vi "Real_time_success.vi"() -> ()   [LabVIEW 2018]
uses:
  <vilib>/Analysis/_algsub.llb/Vector Norm.vi
  <vilib>/Analysis/_algsub.llb/Real Vector Norm.vi
  <vilib>/Analysis/baseanly.llb/Outer Product.vi
  <vilib>/Analysis/baseanly.llb/Real Outer Product.vi
  <vilib>/robotics/Kinematics/Create Lie Group Matrix.vi
  <vilib>/Analysis/baseanly.llb/Real Inverse Matrix.vi
  <vilib>/imath/engines/lvmath2/RunTimeEngine/NodeEndStatement/NIMS_NodeEndStatement_Output.vi
  <instcachedir>/0/NIMS_NodeEndStatement_Output_53EC0D466D134D7ABD903AC30B43404B.lvgen/NIMS_NodeEndStatement_Output_53EC0D466D134D7ABD903AC30B43404B_005.vi
  <instcachedir>/0/NIMS_NodeEndStatement_Output_53EC0D466D134D7ABD903AC30B43404B.lvgen/NIMS_NodeEndStatement_Output_53EC0D466D134D7ABD903AC30B43404B_000.vi
  <instcachedir>/0/NIMS_NodeEndStatement_Output_53EC0D466D134D7ABD903AC30B43404B.lvgen/NIMS_NodeEndStatement_Output_53EC0D466D134D7ABD903AC30B43404B_002.vi
  <vilib>/imath/engines/lvmath2/RunTimeEngine/ErrorHandling/NIMS_Finalize Error.vi
  <vilib>/Analysis/Matrix/Numeric/Conversions/Matrix To Array - RM.vi
  <vilib>/imath/engines/lvmath2/RunTimeEngine/IndexRead/NIMS M(S,S).vi
  <instcachedir>/0/NIMS M(S,S)_AC51E74150A542F7991B9634C66F3096.lvgen/NIMS M(S,S)_AC51E74150A542F7991B9634C66F3096_000.vi
  <vilib>/imath/engines/lvmath2/RunTimeEngine/BuiltInFunctions/abs/NIMS_abs(signed).vi
  <instcachedir>/0/NIMS_abs(signed)_C4FCB8E6058B49B797C7C8D53CA5F6EC.lvgen/NIMS_abs(signed)_C4FCB8E6058B49B797C7C8D53CA5F6EC_000.vi
  <vilib>/imathl/engines/lvmath/Functions/Error Handling/Create Error.vi
  <vilib>/imath/engines/lvmath2/RunTimeEngine/BuiltInFunctions/atan2/NIMS_atan2.vi
  <instcachedir>/0/NIMS_atan2_A91AA4A7D42247EDBE8F76DB99AF04A4.lvgen/NIMS_atan2_A91AA4A7D42247EDBE8F76DB99AF04A4_002.vi
  <vilib>/imath/engines/lvmath2/RunTimeEngine/ErrorHandling/NIMS_Create Error From Enums.vi
  <vilib>/imath/engines/lvmath2/RunTimeEngine/BuiltInFunctions/cos/NIMS_cos(C).vi
  <instcachedir>/0/NIMS_cos(C)_96B8A70E6B8E4D29AD8526A89C8CF3DF.lvgen/NIMS_cos(C)_96B8A70E6B8E4D29AD8526A89C8CF3DF_001.vi
  <instcachedir>/0/NIMS_atan2_A91AA4A7D42247EDBE8F76DB99AF04A4.lvgen/NIMS_atan2_A91AA4A7D42247EDBE8F76DB99AF04A4_001.vi
  <vilib>/imath/engines/lvmath2/RunTimeEngine/IndexRead/NIMS V(S).vi
  <instcachedir>/0/NIMS V(S)_0488751826AF41519A22953C041130DC.lvgen/NIMS V(S)_0488751826AF41519A22953C041130DC_003.vi
  <vilib>/imath/engines/lvmath2/RunTimeEngine/BuiltInFunctions/sin/NIMS_sin(C).vi
  <instcachedir>/0/NIMS_sin(C)_7FE83C8DCD97403BBE687635FA1F837E.lvgen/NIMS_sin(C)_7FE83C8DCD97403BBE687635FA1F837E_001.vi
  <instcachedir>/0/NIMS V(S)_0488751826AF41519A22953C041130DC.lvgen/NIMS V(S)_0488751826AF41519A22953C041130DC_000.vi
  <vilib>/imath/engines/lvmath2/RunTimeEngine/ArithmeticOperatorToken/NIMS_ArithmeticOperator_multmx.vi
  <instcachedir>/0/NIMS_ArithmeticOperator_multmx_622CA76F9646436AB036D42A9A1CE0E6.lvgen/NIMS_ArithmeticOperator_multmx_622CA76F9646436AB036D42A9A1CE0E6_004.vi
  <vilib>/imath/engines/lvmath2/RunTimeEngine/ArithmeticOperatorToken/NIMS_ArithmeticOperator_multmx(M,CV).vi
  <instcachedir>/0/NIMS_ArithmeticOperator_multmx(M,CV)_2F1CD6A2FE4F4213A4AD1C901C2750F5.lvgen/NIMS_ArithmeticOperator_multmx(M,CV)_2F1CD6A2FE4F4213A4AD1C901C2750F5_000.vi
  <vilib>/imath/engines/lvmath2/RunTimeEngine/ArithmeticOperatorToken/NIMS_ArithmeticOperator_multmx(M,CV)-internal.vi
  <instcachedir>/0/NIMS_ArithmeticOperator_multmx(M,CV)-internal_5287250D8D1D4A3E9F77F5DF08D432E0.lvgen/NIMS_ArithmeticOperator_multmx(M,CV)-internal_5287250D8D1D4A3E9F77F5DF08D432E0_004.vi
  <vilib>/imath/engines/lvmath2/RunTimeEngine/ArithmeticOperatorToken/NIMS_ArithmeticOperator_minus.vi
  <instcachedir>/0/NIMS_ArithmeticOperator_minus_C4D0373119CC411691B2E50DF2E09F22.lvgen/NIMS_ArithmeticOperator_minus_C4D0373119CC411691B2E50DF2E09F22_009.vi
  <instcachedir>/0/NIMS_ArithmeticOperator_multmx_622CA76F9646436AB036D42A9A1CE0E6.lvgen/NIMS_ArithmeticOperator_multmx_622CA76F9646436AB036D42A9A1CE0E6_008.vi
  <vilib>/imath/engines/lvmath2/RunTimeEngine/IndexRead/NIMS M(S).vi
  <instcachedir>/0/NIMS M(S)_B826C018497E4940AE96BD27B540B6FB.lvgen/NIMS M(S)_B826C018497E4940AE96BD27B540B6FB_004.vi
  <vilib>/imath/engines/lvmath2/RunTimeEngine/Managers/WorkSpace/UID Generator.vi
  <vilib>/imath/engines/lvmath2/RunTimeEngine/RunTimeType/NIMS_RunTimeType_From StrictType (excl LVString).vi
  <instcachedir>/0/NIMS_RunTimeType_From StrictType (excl LVString)_E7E34A65C99947108168652BAD14964D.lvgen/NIMS_RunTimeType_From StrictType (excl LVString)_E7E34A65C99947108168652BAD14964D_000.vi
  <vilib>/imath/engines/lvmath2/RunTimeEngine/LocalVariableDefStatement/MC_LocalVariableDefStatement_Display.vi
  <instcachedir>/0/NIMS M(S)_B826C018497E4940AE96BD27B540B6FB.lvgen/NIMS M(S)_B826C018497E4940AE96BD27B540B6FB_000.vi
  <vilib>/imath/engines/lvmath2/RunTimeEngine/Managers/SymbolTable/Clear UID.vi
  <vilib>/Analysis/Matrix/Numeric/Multiply/Multiply.vi
  <vilib>/Analysis/Matrix/Numeric/Multiply/Multiply - RM,R.vi
  <vilib>/Analysis/Matrix/Numeric/Multiply/Multiply - R,RM.vi
  <vilib>/Analysis/Matrix/Numeric/Add/Add.vi
  <vilib>/Analysis/Matrix/Numeric/Add/Add - RM,RM.vi
  <instcachedir>/0/NIMS_NodeEndStatement_Output_53EC0D466D134D7ABD903AC30B43404B.lvgen/NIMS_NodeEndStatement_Output_53EC0D466D134D7ABD903AC30B43404B_001.vi
  <instcachedir>/0/NIMS_NodeEndStatement_Output_53EC0D466D134D7ABD903AC30B43404B.lvgen/NIMS_NodeEndStatement_Output_53EC0D466D134D7ABD903AC30B43404B_008.vi
  <vilib>/imath/engines/lvmath2/RunTimeEngine/IndexRead/NIMS M($,S).vi
  <instcachedir>/0/NIMS M($,S)_3E5749BBB62E49528D4765A77F1F6D98.lvgen/NIMS M($,S)_3E5749BBB62E49528D4765A77F1F6D98_000.vi
  <vilib>/imath/engines/lvmath2/RunTimeEngine/RowToken/NIMS_RowToken_SorRV_CV.vi
  <instcachedir>/0/NIMS_RowToken_SorRV_CV_E9A223509C5746E8B9F22970C86A52C1.lvgen/NIMS_RowToken_SorRV_CV_E9A223509C5746E8B9F22970C86A52C1_000.vi
  <vilib>/Analysis/NI_AALBase.lvlib
  <vilib>/gmath/NI_Gmath.lvlib
  <vilib>/Analysis/Matrix/NI_Matrix.lvlib
  <vilib>/robotics/Kinematics/NI_Kinematics.lvlib
  <vilib>/imath/engines/lvmath2/RunTimeEngine/Managers/SymbolTable/NIMS_WorkSpace.lvlib
panel:
  out "Yaw":cluster{"E1_now":dbl[], "t_now":dbl[]}(graph)
  out "Pitch":cluster{"E1_now":dbl[], "t_now":dbl[]}(graph)
  out "Roll":cluster{"E1_now":dbl[], "t_now":dbl[]}(graph)
  in  "MOI(kg*m^2)":dbl[][](array[numeric])
  in  "COG(m)":dbl[](array[numeric])
  in  "Mass (kg)":dbl
  in  "Simulation Time(sec)":dbl
  # "Physical Parameters"
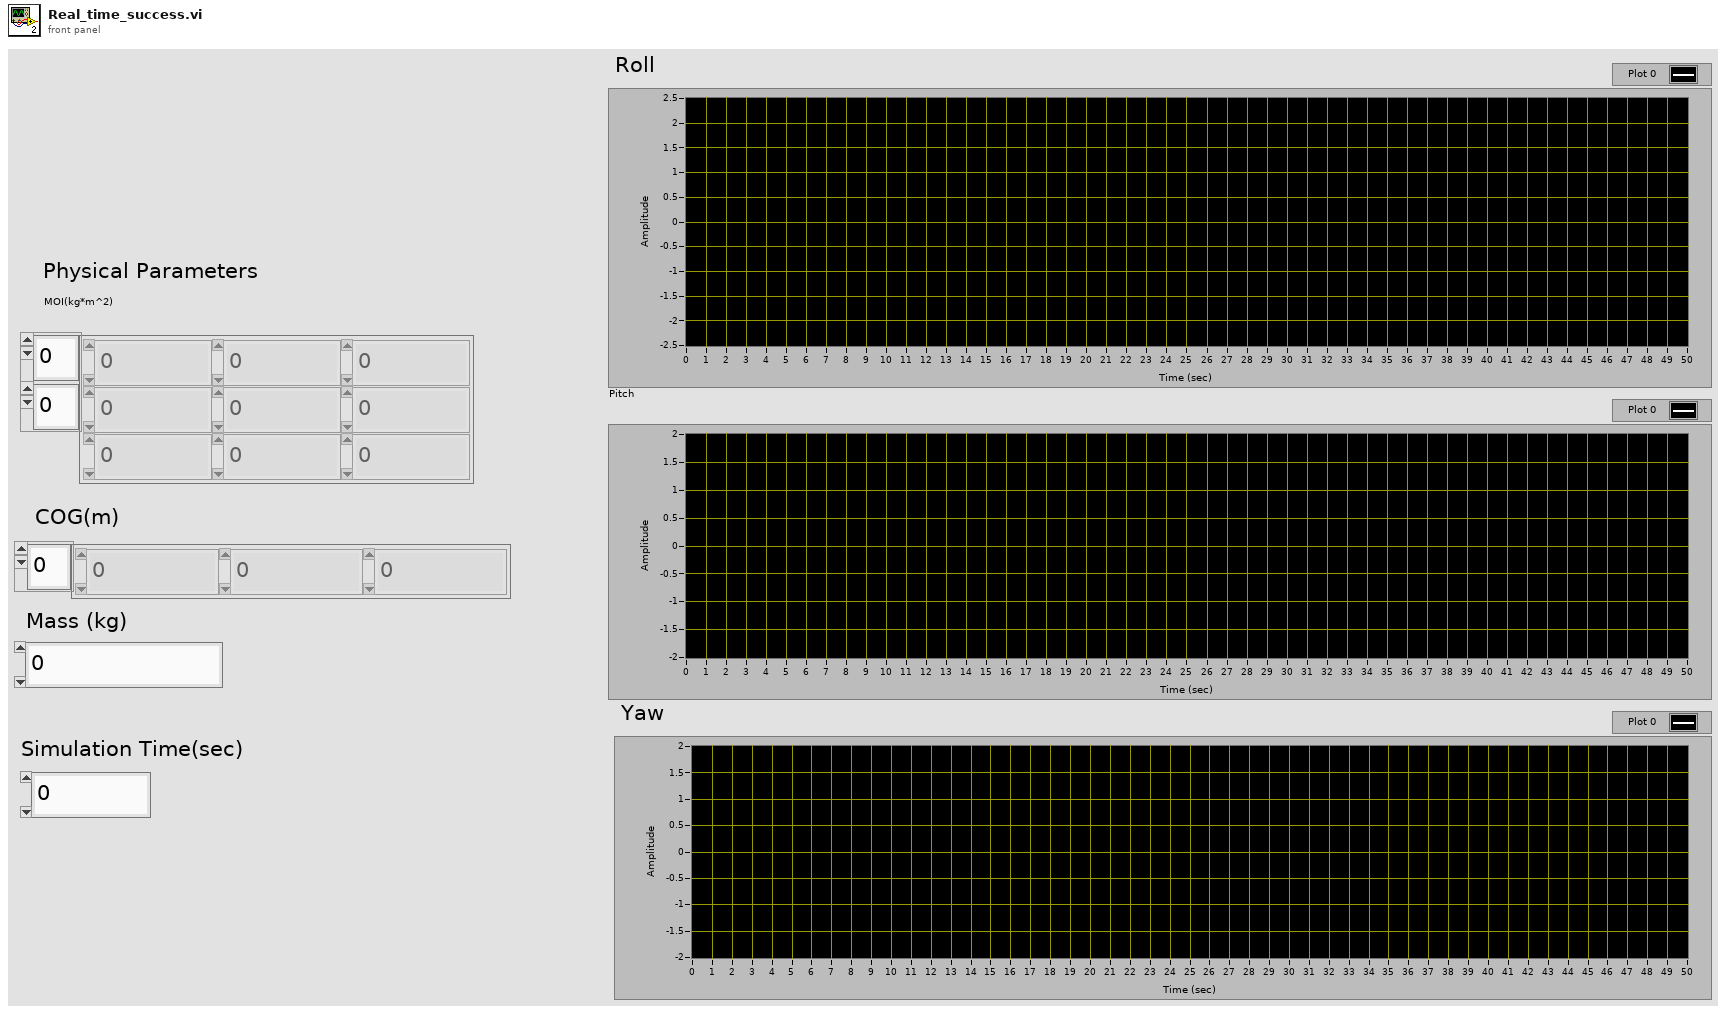
[diagram p1: front panel]
types:
  T1 = cluster{"E1":cdb[], "E2":dbl[], "E3":dbl[], "t":dbl[]}
  T2 = typedef "NI_Matrix.lvlib/RealMatrix.ctl" = dbl[][]
  T3 = typedef "NI_Kinematics.lvlib/Quaternion.ctl" = dbl[]
  T4 = cluster{"E1_now":cdb[], "E2_now":cdb[], "E3_now":dbl[], "t_now":dbl[]}
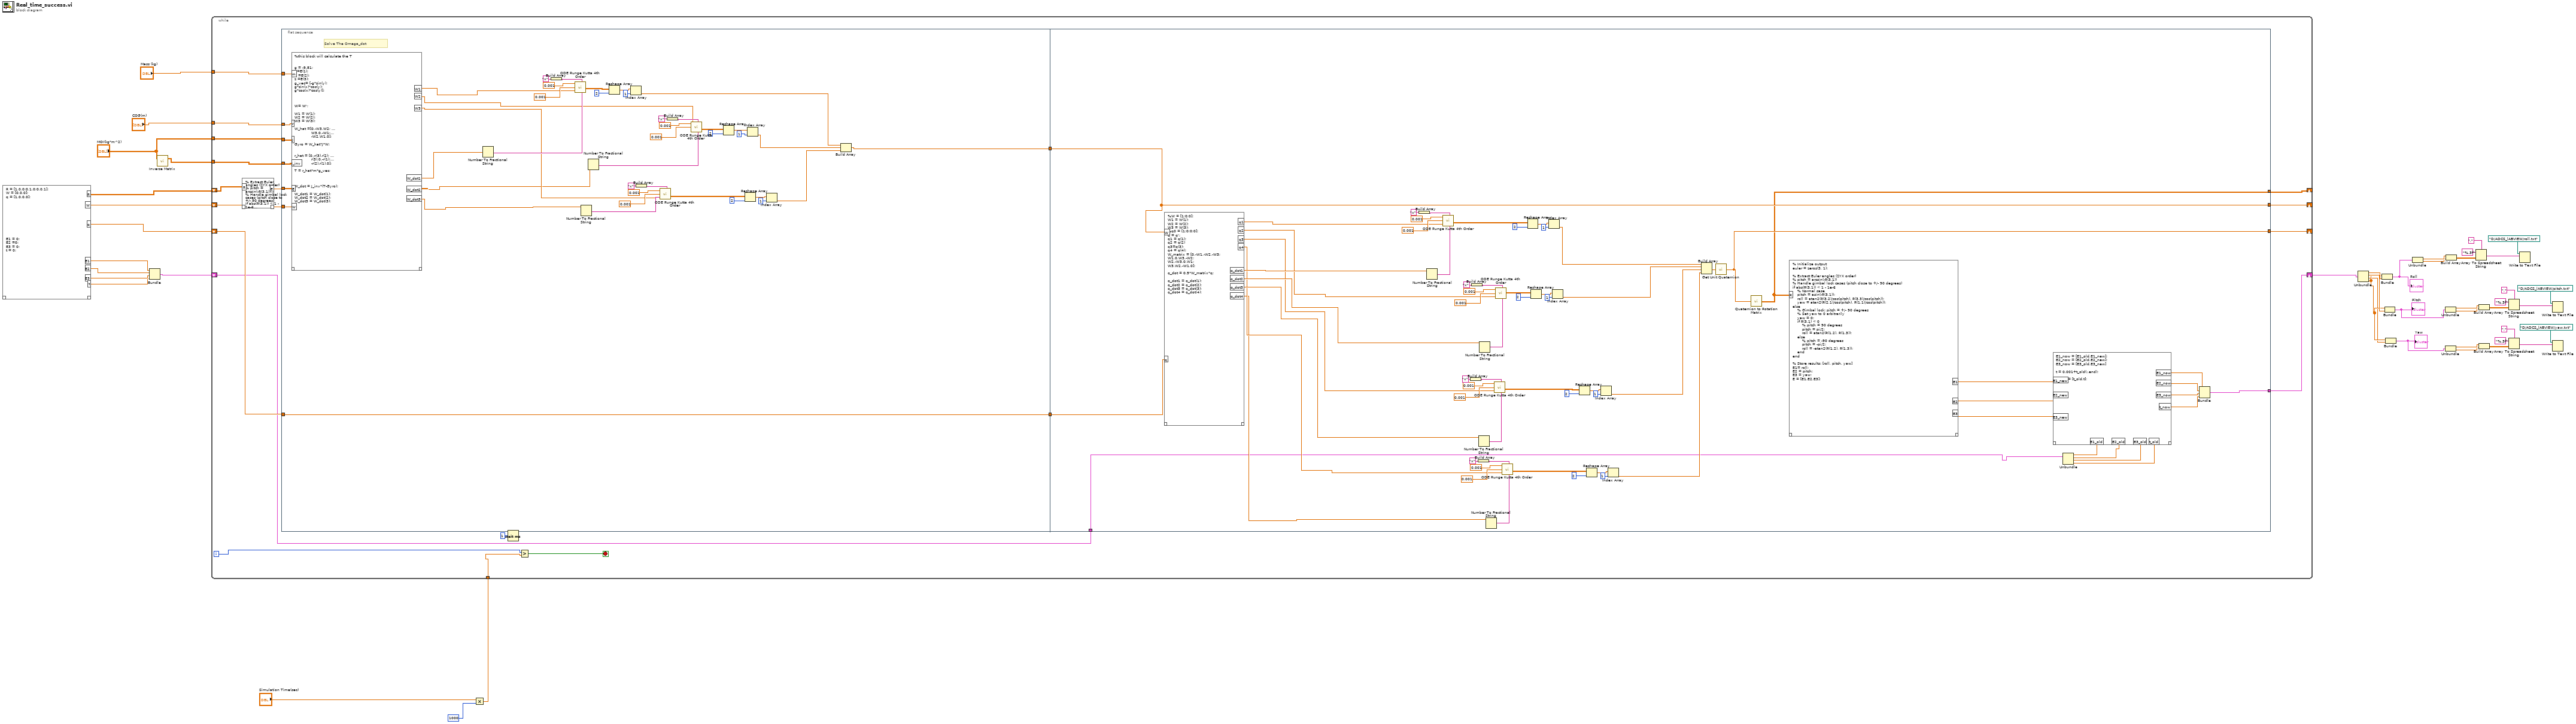
[diagram p0: block diagram]
diagram:
  n1 = mathscript code="R = [1,0,0;0,1,0;0,0,1];\nW = [0,0,0];\nq = [1,0,0,0];\n\n\n\n\n\n\n\n\n\n\nE1 = 0;\nE2 =0;\nE3 = 0;\nt = 0;"() -> ("R"=w37:dbl[][], "W"=w36:dbl[], "q"=w35:dbl[], "E1"=w34:cdb[], "E2"=w33:dbl[], "E3"=w32:dbl[], "t"=w30:dbl[])  [unwired: 1 in, 1 out]
  n2 = Bundle("E1"=w34, "E2"=w33, "E3"=w32, "t"=w30) -> (w31:T1)  [unwired: 1 in]
  n3 = call-poly <vilib>:"Inverse Matrix.vi"("Input Matrix"="MOI(kg*m^2)") -> ("Inverse Matrix"=w39:T2)  [unwired: 1 in, 1 out]
  n4 = Multiply(x="Simulation Time(sec)", y=1000) -> (x*y=w42:dbl)
  n5 = while {
    tunnel: w42 -> [w49]
    tunnel: "Mass (kg)" -> [w59]
    tunnel: "COG(m)" -> [w60]
    tunnel: w39 -> [w62]
    tunnel: "MOI(kg*m^2)" -> [w61]
    shift-right: [w52] -> _
    shift-left: w37 -> [w57]
    shift-right: [w51] -> _
    shift-left: w36 -> [w58]
    shift-right: [w53] -> _
    shift-left: w35 -> [w54]
    shift-right: [w46] -> w29
    shift-left: w31 -> [w47]
    i -> [w48]
    stop <- w50 stop-if-true
    n6 = mathscript code="% Extract Euler angles (ZYX order)\n% pitch = arcsin(-R(3,1))\n% Handle gimbal lock cases (pitch close to +/- 90 degrees)\nif abs(R(3,1)) < 1 - 1e-6\n    % Normal case\n    pitch = asin(-R(3,1));\n    roll = atan2(R(3,2)/cos(pitch), R(3,3)/cos(pitch));\n    yaw = atan2(R(2,1)/cos(pitch), R(1,1)/cos(pitch));\nelse\n    % Gimbal lock: pitch = +/- 90 degrees\n    % Set yaw to 0 arbitrarily\n    yaw = 0;\n    if R(3,1) < 0\n        % pitch = 90 degrees\n        pitch = pi/2;\n        roll = atan2(R(1,2), R(1,3));\n    else\n        % pitch = -90 degrees\n        pitch = -pi/2;\n        roll = -atan2(R(1,2), R(1,3));\n    end\nend\n\n% Store results: [roll, pitch, yaw]\nE1= roll;\nE2 = pitch;\nE3 = yaw;\nE = [E1,E2,E3];"("R"=w57) -> ("E"=w56:cdb[])  [unwired: 1 in, 1 out]
    n7 = flat-sequence {
      tunnel: w56 -> [w383]
      tunnel: w62 -> [w382]
      tunnel: w61 -> [w381]
      tunnel: w60 -> [w380]
      tunnel: w59 -> [w379]
      tunnel: w58 -> [w378]
      tunnel: [w341] -> w55
      tunnel: w54 -> [w341]
      tunnel: [w340] -> w45
      tunnel: w55 -> [w803]
      tunnel: [w802] -> w53
      tunnel: [w800] -> w52
      tunnel: [w801] -> w51
      tunnel: w47 -> [w793]
      tunnel: [w789] -> w46
      tunnel: w45 -> [w801]
      frame #0 {
        # "Solve The Omega_dot"
        n8 = mathscript code="%this block will calculate the T\n\n\ng = -9.81;\nx=E(1);\ny =E(2);\nz =E(3);\ng_vec= [-g*sin(y);\ng*sin(x)*cos(y);\ng*cos(x)*cos(y)];\n\n\n\nW= W';\n\nW1 = W(1);\nW2 = W(2);\nW3 = W(3);\n\nW_hat =[0,-W3,W2; ...\n              W3,0,-W1;...\n              -W2,W1,0];\n\nGyro = W_hat*J*W;\n\n\nr_hat = [0,-r(3),r(2); ...\n              r(3),0,-r(1);...\n              -r(2),r(1),0];\n\nT = r_hat*m*g_vec;\n\n\n\nW_dot = J_inv*(T-Gyro);\n\nW_dot1 = W_dot(1);\nW_dot2 = W_dot(2);\nW_dot3 = W_dot(3);"("E"=w383, "J"=w381, "J_inv"=w382, "r"=w380, "m"=w379, "W"=w378) -> ("W_dot1"=w342:dbl[], "W_dot2"=w343:dbl[], "W_dot3"=w344:dbl[], "W1"=w347:dbl[], "W2"=w346:dbl[], "W3"=w345:dbl[])  [unwired: 1 in, 1 out]
        n9 = Number To Fractional String(number=w342) -> (F-format string=w373:string[])  [unwired: 3 in]
        n10 = Build Array("x") -> (w376:string[])
        n11 = call <vilib>:"ODE Runge Kutta 4th Order.vi"("time end"=0.001, "h (step rate)"=0.001, "X0"=w347, "X (name of variables)"=w376, "F(X,t) (right sides of the ODE\nas functions of X and t)"=w373) -> ("X Values (solution)"=w369:dbl[][])  [unwired: 2 in, 3 out]
        n12 = Number To Fractional String(number=w344) -> (F-format string=w355:string[])  [unwired: 3 in]
        n13 = Number To Fractional String(number=w343) -> (F-format string=w364:string[])  [unwired: 3 in]
        n14 = Reshape Array(w369, 2 ("dimension size")) -> (w371:dbl[])
        n15 = Index Array(array=w371, index=1) -> (element=w350:dbl)
        n16 = Build Array("x") -> (w358:string[])
        n17 = call <vilib>:"ODE Runge Kutta 4th Order.vi"("time end"=0.001, "h (step rate)"=0.001, "X0"=w345, "X (name of variables)"=w358, "F(X,t) (right sides of the ODE\nas functions of X and t)"=w355) -> ("X Values (solution)"=w351:dbl[][])  [unwired: 2 in, 3 out]
        n18 = Build Array("x") -> (w367:string[])
        n19 = call <vilib>:"ODE Runge Kutta 4th Order.vi"("time end"=0.001, "h (step rate)"=0.001, "X0"=w346, "X (name of variables)"=w367, "F(X,t) (right sides of the ODE\nas functions of X and t)"=w364) -> ("X Values (solution)"=w360:dbl[][])  [unwired: 2 in, 3 out]
        n20 = Reshape Array(w360, 2 ("dimension size")) -> (w362:dbl[])
        n21 = Reshape Array(w351, 2 ("dimension size")) -> (w353:dbl[])
        n22 = Index Array(array=w362, index=1) -> (element=w349:dbl)
        n23 = Index Array(array=w353, index=1) -> (element=w348:dbl)
        n24 = Build Array(w350, w349, w348) -> (w340:dbl[])
      }
      frame #1 {
        n25 = mathscript code="%W = [1;0;0];\nW1 = W(1);\nW2 = W(2);\nW3 = W(3);\n%q0 = [1;0;0;0];\nq = q';\nq1 = q(1);\nq2 = q(2)\nq3=q(3);\nq4 = q(4);\nW_matrix = [0,-W1,-W2,-W3;\nW1,0,W3,-W2;\nW2,-W3,0,W1;\nW3,W2,-W1,0];\n\nq_dot = 0.5*W_matrix*q;\n\nq_dot1 = q_dot(1);\nq_dot2 = q_dot(2);\nq_dot3 = q_dot(3);\nq_dot4 = q_dot(4);"("q"=w803, "W"=w801) -> ("q_dot1"=w842:dbl[], "q_dot2"=w831:dbl[], "q_dot3"=w820:dbl[], "q_dot4"=w809:dbl[], "q1"=w843:dbl[], "q2"=w832:dbl[], "q3"=w821:dbl[], "q4"=w810:dbl[])  [unwired: 1 in, 1 out]
        n26 = Build Array("x") -> (w851:string[])
        n27 = Number To Fractional String(number=w842) -> (F-format string=w848:string[])  [unwired: 3 in]
        n28 = call <vilib>:"ODE Runge Kutta 4th Order.vi"("time end"=0.001, "h (step rate)"=0.001, "X0"=w843, "X (name of variables)"=w851, "F(X,t) (right sides of the ODE\nas functions of X and t)"=w848) -> ("X Values (solution)"=w844:dbl[][])  [unwired: 2 in, 3 out]
        n29 = Build Array("x") -> (w829:string[])
        n30 = Build Array("x") -> (w840:string[])
        n31 = Build Array("x") -> (w818:string[])
        n32 = Number To Fractional String(number=w820) -> (F-format string=w826:string[])  [unwired: 3 in]
        n33 = Number To Fractional String(number=w831) -> (F-format string=w837:string[])  [unwired: 3 in]
        n34 = Number To Fractional String(number=w809) -> (F-format string=w815:string[])  [unwired: 3 in]
        n35 = call <vilib>:"ODE Runge Kutta 4th Order.vi"("time end"=0.001, "h (step rate)"=0.001, "X0"=w821, "X (name of variables)"=w829, "F(X,t) (right sides of the ODE\nas functions of X and t)"=w826) -> ("X Values (solution)"=w822:dbl[][])  [unwired: 2 in, 3 out]
        n36 = call <vilib>:"ODE Runge Kutta 4th Order.vi"("time end"=0.001, "h (step rate)"=0.001, "X0"=w832, "X (name of variables)"=w840, "F(X,t) (right sides of the ODE\nas functions of X and t)"=w837) -> ("X Values (solution)"=w833:dbl[][])  [unwired: 2 in, 3 out]
        n37 = call <vilib>:"ODE Runge Kutta 4th Order.vi"("time end"=0.001, "h (step rate)"=0.001, "X0"=w810, "X (name of variables)"=w818, "F(X,t) (right sides of the ODE\nas functions of X and t)"=w815) -> ("X Values (solution)"=w811:dbl[][])  [unwired: 2 in, 3 out]
        n38 = Reshape Array(w844, 2 ("dimension size")) -> (w846:dbl[])
        n39 = Reshape Array(w833, 2 ("dimension size")) -> (w835:dbl[])
        n40 = Index Array(array=w846, index=1) -> (element=w808:dbl)
        n41 = Index Array(array=w835, index=1) -> (element=w807:dbl)
        n42 = Reshape Array(w822, 2 ("dimension size")) -> (w824:dbl[])
        n43 = Reshape Array(w811, 2 ("dimension size")) -> (w813:dbl[])
        n44 = Index Array(array=w824, index=1) -> (element=w806:dbl)
        n45 = Index Array(array=w813, index=1) -> (element=w805:dbl)
        n46 = Build Array(w808, w807, w806, w805) -> (w804:dbl[])
        n47 = call <vilib>:"Get Unit Quaternion.vi"("quaternion"=w804) -> ("unit quaternion"=w802:T3)
        n48 = call <vilib>:"Quaternion to Rotation Matrix.vi"("quaternion"=w802) -> ("rotation matrix"=w800:T2)
        n49 = mathscript code="% Initialize output\neuler = zeros(3, 1);\n\n% Extract Euler angles (ZYX order)\n% pitch = arcsin(-R(3,1))\n% Handle gimbal lock cases (pitch close to +/- 90 degrees)\nif abs(R(3,1)) < 1 - 1e-6\n    % Normal case\n    pitch = asin(-R(3,1));\n    roll = atan2(R(3,2)/cos(pitch), R(3,3)/cos(pitch));\n    yaw = atan2(R(2,1)/cos(pitch), R(1,1)/cos(pitch));\nelse\n    % Gimbal lock: pitch = +/- 90 degrees\n    % Set yaw to 0 arbitrarily\n    yaw = 0;\n    if R(3,1) < 0\n        % pitch = 90 degrees\n        pitch = pi/2;\n        roll = atan2(R(1,2), R(1,3));\n    else\n        % pitch = -90 degrees\n        pitch = -pi/2;\n        roll = -atan2(R(1,2), R(1,3));\n    end\nend\n\n% Store results: [roll, pitch, yaw]\nE1= roll;\nE2 = pitch;\nE3 = yaw;\nE = [E1,E2,E3];"("R"=w800) -> ("E1"=w799:dbl, "E2"=w798:cdb, "E3"=w797:dbl)  [unwired: 1 in, 1 out]
        n50 = Unbundle(w793) -> ("E1_now"=w796:cdb[], "E2_now"=w795:cdb[], "E3_now"=w794:dbl[], "t_now"=w787:dbl[])
        n51 = mathscript code="E1_now = [E1_old,E1_new];\nE2_now = [E2_old,E2_new];\nE3_now = [E3_old,E3_new]\n\nt = 0.001+t_old(:,end);\n\nt_now = [t_old,t];"("E1_new"=w799, "E2_new"=w798, "E3_new"=w797, "E1_old"=w796, "E2_old"=w795, "E3_old"=w794, "t_old"=w787) -> ("E1_now"=w792:cdb[], "E2_now"=w791:cdb[], "E3_now"=w790:dbl[], "t_now"=w788:dbl[])  [unwired: 1 in, 1 out]
        n52 = Bundle("E1_now"=w792, "E2_now"=w791, "E3_now"=w790, "t_now"=w788) -> (w789:T4)  [unwired: 1 in]
      }
    }
    n53 = Wait (ms)(milliseconds to wait=u32 1) -> ()  [unwired: 1 out]
    n54 = Greater?(x=w48, y=w49) -> (0:w50:bool)
  }
  n55 = Unbundle(w29) -> ("E1_now"=w28:cdb[], "E2_now"=w27:cdb[], "E3_now"=w25:dbl[], "t_now"=w26:dbl[])
  n56 = Bundle("t_now"=w26, "E1_now"=w28) -> (w24:cluster{"t_now":dbl[], "E1_now":cdb[]})  [unwired: 1 in]
  "Roll" <- w24
  n57 = Bundle("t_now"=w26, "E2_now"=w27) -> (w9:cluster{"t_now":dbl[], "E2_now":cdb[]})  [unwired: 1 in]
  "Pitch" <- w9
  n58 = Bundle("t_now"=w26, "E3_now"=w25) -> (w1:cluster{"t_now":dbl[], "E3_now":dbl[]})  [unwired: 1 in]
  "Yaw" <- w1
  n59 = Unbundle(w24) -> ("t_now"=w23:dbl[], "E1_now"=w22:cdb[])
  n60 = Unbundle(w9) -> ("t_now"=w16:dbl[], "E2_now"=w15:cdb[])
  n61 = Unbundle(w1) -> ("t_now"=w8:dbl[], "E3_now"=w7:dbl[])
  n62 = Build Array(w23, w22) -> (w21:cdb[][])
  n63 = Array To Spreadsheet String(delimiter (Tab)=",", array=w21, 3:"%.3f" ("format string")) -> (spreadsheet string=w18:string)
  n64 = Build Array(w16, w15) -> (w14:cdb[][])
  n65 = Build Array(w8, w7) -> (w6:dbl[][])
  n66 = Array To Spreadsheet String(delimiter (Tab)=",", array=w14, 3:"%.3f" ("format string")) -> (spreadsheet string=w11:string)
  n67 = Array To Spreadsheet String(delimiter (Tab)=",", array=w6, 3:"%.3f" ("format string")) -> (spreadsheet string=w3:string)
  n68 = Write to Text File(file (use dialog)=path "D:/ADCS_lABVIEW/roll.txt", text=w18) -> ()  [unwired: 2 in, 3 out]
  n69 = Write to Text File(file (use dialog)=path "D:/ADCS_lABVIEW/pitch.txt", text=w11) -> ()  [unwired: 2 in, 3 out]
  n70 = Write to Text File(file (use dialog)=path "D:/ADCS_lABVIEW/yaw.txt", text=w3) -> ()  [unwired: 2 in, 3 out]
